vi "Calc_Conc.vi"(1 "Extinction (cm-1)":dbl[](array[numeric]), 4 "Pressure":dbl, 6 "Temperature":dbl) -> (21 "NO2 Conc (ppb)":dbl, 25 "Gly Conc (ppb)":dbl)   [LabVIEW 2025]
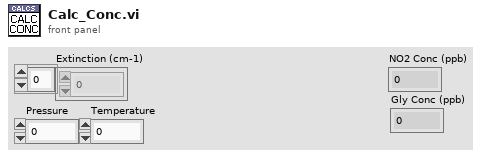
[diagram p1: front panel]
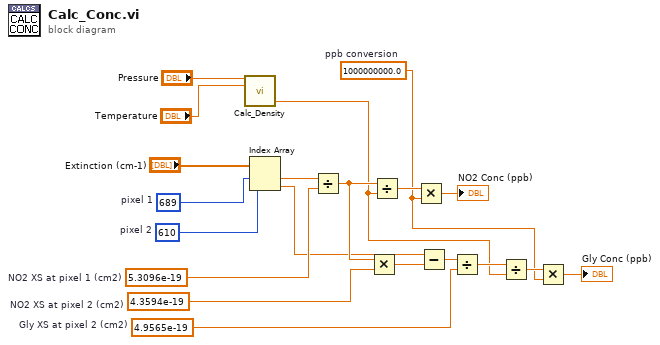
[diagram p0: block diagram]
diagram:
  w18 = 610  # pixel 2
  w19 = 689  # pixel 1
  w10 = 4.3594e-19  # NO2 XS at pixel 2 (cm2)
  w2 = 1000000000.0  # ppb conversion
  w6 = 4.9565e-19  # Gly XS at pixel 2 (cm2)
  w17 = 5.3096e-19  # NO2 XS at pixel 1 (cm2)
  n1 = call "Calc_Density.vi"("Pres (hPa)"="Pressure", "T (C)"="Temperature") -> ("Density (cm^-3)"=w4:dbl)  [unwired: 25 in]
  n2 = Index Array(array="Extinction (cm-1)", index #1=w19, index #2=w18) -> (element #1=w12:dbl, element #2=w8:dbl)
  n3 = Divide(x=w12, y=w17) -> (x/y=w11:dbl)
  n4 = Multiply(x=w11, y=w10) -> (x*y=w9:dbl)
  n5 = Divide(x=w11, y=w4) -> (x/y=w14:dbl)
  n6 = Multiply(x=w14, y=w2) -> (x*y=→"NO2 Conc (ppb)":dbl)
  n7 = Subtract(x=w8, y=w9) -> (x-y=w7:dbl)
  n8 = Divide(x=w7, y=w6) -> (x/y=w5:dbl)
  n9 = Divide(x=w5, y=w4) -> (x/y=w3:dbl)
  n10 = Multiply(x=w3, y=w2) -> (x*y=→"Gly Conc (ppb)":dbl)
